vi "RT Shared Binary Path.vi"() -> (0 "Path":path)   [LabVIEW 2020]
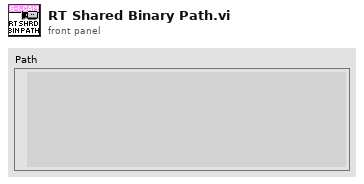
[diagram p1: front panel]
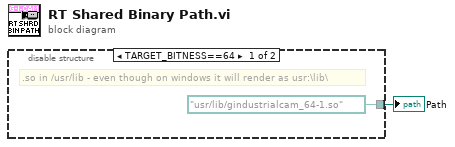
[diagram p0: block diagram]
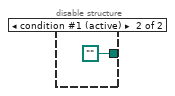
[diagram p2: hidden frame]
diagram:
  n1 = disable-structure shown="TARGET_BITNESS==64" {
    disable-tunnel: [path "/usr/lib/gindustrialcam_64-1.so" path "" ("Path")] -> w1
    frame condition #0 {
      # ".so in /usr/lib - even though on windows it will render as usr:\\lib\\"
    }
    frame condition #1 (active) {
    }
  }
  "Path" <- w1
